vi "tagDB_Obtain.vi"(4 "error in (no error)":errorcluster, 7 "name (unnamed)":string) -> (0 "error out":errorcluster, 1 "created new":bool, 3 "DB":T1)   [LabVIEW 2014, in "TagDB(dev).lvlib"]
doc: "[Covers: REQ_API_Obtain]"
uses:
  TagDB(dev).lvlib
  tagDB_Def.ctl
  _Support/Private/_DEF-DBOper.ctl
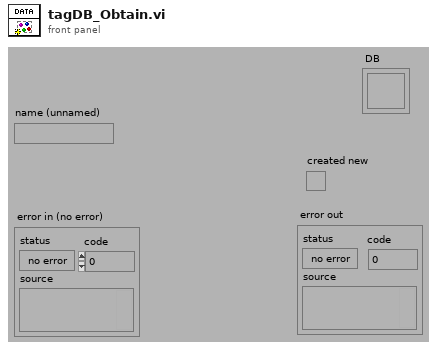
[diagram p1: front panel]
types:
  T1 = typedef "TagDB(dev).lvlib/tagDB_Def.ctl" = refnum<k1>
  T2 = typedef "TagDB(dev).lvlib/_DEF-DBOper.ctl" = enum16{"create", "destroy", "cleanUp", "list", "get info"}
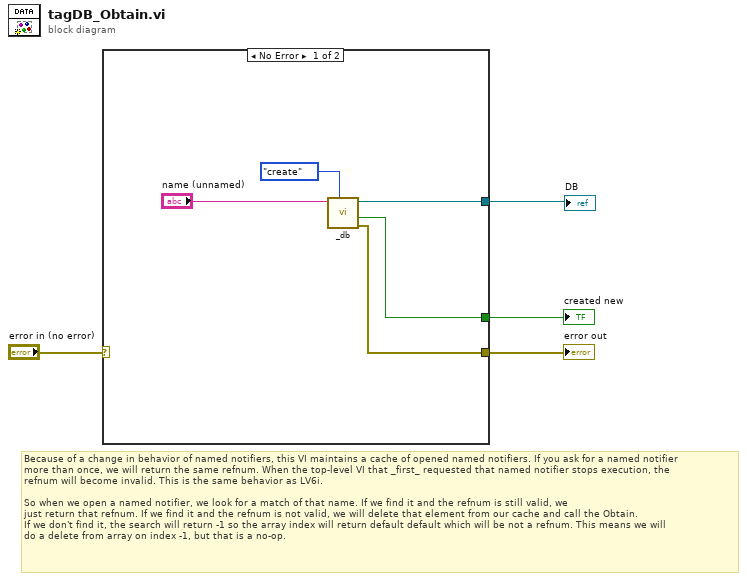
[diagram p0: block diagram]
diagram:
  # "Because of a change in behavior of named notifiers, this VI maintains a cache of opened named notifiers. If you ask for a named notifier\nmore than once, we will return the same refnum. When the top-level VI that _first_ requested that named notifier stops execution, the\nrefnum will become invalid. This is the same behavior as LV6i.\n\nSo when we open a named notifier, we look for a match of that name. If we find it and the refnum is still valid, we\njust return that refnum. If we find it and the refnum is not valid, we will delete that element from our cache and call the Obtain.\nIf we don't find it, the search will return -1 so the array index will return default default which will be not a refnum. This means we will\ndo a delete from array on index -1, but that is a no-op."
  n1 = case shown="No Error" "error in (no error)" {
    selector: "error in (no error)" -> [_ w10]
    tunnel: [w7 w10] -> w4
    tunnel: [w6 _] -> w3
    tunnel: [w8 _] -> w2
    frame No Error {
      n2 = call "_db.vi"("command"=_DEF-DBOper."create", "name"="name (unnamed)") -> ("error out"=w7:errorcluster, "created new?"=w6:bool, "db out"=w8:T1)  [unwired: 5 in, 2 out]
    }
    frame Error {
    }
  }
  "error out" <- w4
  "created new" <- w3
  "DB" <- w2
